vi "WordW.vi"() -> ()   [LabVIEW 2018]
uses:
  <vilib>/Utility/file.llb/Read Delimited Spreadsheet (DBL).vi
panel:
  out "all rows":dbl[][](array[numeric])=[[-3.0, 2.5, -0.75], [-2.99997, 2.50243, -0.75116], [-2.99977, 2.5097, -0.75467], [-2.99909, 2.52168, -0.76053], [-2.99738, 2.53817, -0.76879], [-2.99377, 2.55886, -0.77951], [-2.98699, 2.58327, -0.79277], [-2.97521, 2.61077, -0.80868], [-2.95578, 2.64042, -0.82736], [-2.92492, 2.67088, -0.84901], [-2.87757, 2.70007, -0.87371], [-2.81238, 2.72392, -0.89977], [-2.72784, 2.74059, -0.92672], [-2.62235, 2.7491, -0.95466], [-2.49582, 2.74876, -0.98376], [-2.35017, 2.73927, -1.01419], [-2.18926, 2.72078, -1.04619], [-2.01814, 2.6938, -1.08006], [-1.84203, 2.65898, -1.11624], [-1.66534, 2.61696, -1.15531], [-1.49497, 2.56935, -1.19717], [-1.3445, 2.52103, -1.23909], [-1.21356, 2.47381, -1.28087], [-1.10019, 2.42885, -1.32252], [-1.00244, 2.38706, -1.36406], [-0.91853, 2.34919, -1.40552], [-0.847, 2.31588, -1.4469], [-0.78669, 2.28768, -1.48823], [-0.73668, 2.2651, -1.52952], [-0.69628, 2.24858, -1.57079], [-0.69628, 2.24858, -1.57079], [-0.71986, 2.25281, -1.5708], [-0.79005, 2.26256, -1.5708], [-0.90387, 2.26885, -1.5708], [-1.03187, 2.25981, -1.5708], [-1.14644, 2.23301, -1.5708], [-1.24441, 2.18937, -1.5708], [-1.31211, 2.14105, -1.5708], [-1.34651, 2.10717, -1.5708], [-1.35695, 2.0951, -1.5708], [-1.35695, 2.0951, -1.5708], [-1.33968, 2.09833, -1.57079], [-1.28598, 2.10533, -1.57079], [-1.19109, 2.10788, -1.57079], [-1.07045, 2.09589, -1.57079], [-0.94532, 2.06777, -1.57079], [-0.81837, 2.0241, -1.57079], [-0.71267, 1.97638, -1.57079], [-0.64964, 1.943, -1.57079], [-0.62872, 1.9311, -1.57079], [-0.62872, 1.9311, -1.57079], [-0.64677, 1.93354, -1.5708], [-0.69993, 1.93831, -1.5708], [-0.78456, 1.93774, -1.5708], [-0.87807, 1.92299, -1.5708], [-0.96104, 1.8931, -1.5708], [-1.03201, 1.8484, -1.5708], [-1.08123, 1.80008, -1.5708], [-1.10628, 1.76634, -1.57079], [-1.11387, 1.7543, -1.57079], [-1.11387, 1.7543, -1.57079], [-1.09963, 1.75609, -1.57079], [-1.05553, 1.75898, -1.57079], [-0.97789, 1.75558, -1.57079], [-0.87895, 1.73796, -1.57079], [-0.77506, 1.70562, -1.57079], [-0.66745, 1.65865, -1.57079], [-0.57557, 1.6083, -1.57079], [-0.51962, 1.57314, -1.57079], [-0.50084, 1.56059, -1.57079], [-0.50084, 1.56059, -1.57079], [-0.50084, 1.56059, -1.56133], [-0.50084, 1.56059, -1.50808], [-0.50084, 1.56059, -1.39853], [-0.50084, 1.56059, -1.24519], [-0.50084, 1.56059, -1.0756], [-0.50084, 1.56059, -0.92227], [-0.50084, 1.56059, -0.81272], [-0.50084, 1.56059, -0.75947], [-0.50084, 1.56059, -0.75], [-0.50084, 1.56059, -0.75], [-0.50181, 1.56096, -0.75], [-0.50821, 1.56336, -0.75], [-0.52439, 1.56944, -0.75], [-0.5536, 1.58042, -0.75], [-0.59808, 1.59714, -0.75], [-0.65917, 1.62011, -0.75], [-0.73734, 1.64949, -0.75], [-0.83235, 1.6852, -0.75], [-0.94327, 1.7269, -0.75], [-1.06863, 1.77402, -0.75], [-1.20646, 1.82583, -0.75], [-1.35439, 1.88143, -0.75], [-1.50977, 1.93984, -0.75], [-1.66969, 1.99995, -0.75], [-1.83115, 2.06064, -0.75], [-1.99107, 2.12075, -0.75], [-2.14644, 2.17916, -0.75], [-2.29438, 2.23476, -0.75], [-2.43221, 2.28657, -0.75], [-2.55757, 2.33369, -0.75], [-2.66849, 2.37539, -0.75], [-2.7635, 2.4111, -0.75], [-2.84167, 2.44048, -0.75], [-2.90275, 2.46345, -0.75], [-2.94724, 2.48017, -0.75], [-2.97645, 2.49115, -0.75], [-2.99263, 2.49723, -0.75], [-2.99903, 2.49963, -0.75], [-3.0, 2.5, -0.75]]
  in  "file path (dialog if empty)":path=path "/Users/JoshEtkind/Documents/Tufts/Senior Fall/Advanced Robotics/Initials/Physical Robot/wordW.csv"
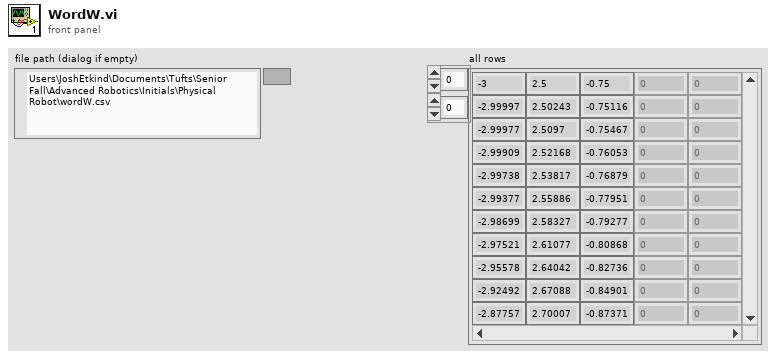
[diagram p1: front panel]
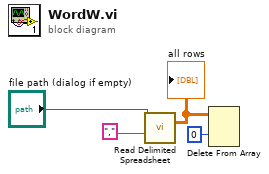
[diagram p0: block diagram]
diagram:
  n1 = call-poly <vilib>:"Read Delimited Spreadsheet.vi"("file path (dialog if empty)"="file path (dialog if empty)", "delimiter (\\t)"="," ("delimiter (\\t)")) -> ("all rows"=w2:dbl[][])  [unwired: 8 in, 5 out]
  "all rows" <- w2
  n2 = Delete From Array(array=w2, index (row)=0) -> ()  [unwired: 2 in, 2 out]
